vi "SwitchingCommand.vi"(9 "command":i32(ring)=1 items=["Cycle"=1, "Step"=2, "Continue"=3], 10 "HighSpeedEServer":refnum<k24>, 11 "error in (no error)":errorcluster) -> (3 "error out":errorcluster)   [LabVIEW 2021, in "UnderAutomation.Yaskawa.lvlib"]
uses:
  UnderAutomation.Yaskawa.lvlib
  C:/Users/fg/Documents/Yaskawa.vi/LabVIEW_2024/UnderAutomation.Yaskawa/lib/UnderAutomation.Yaskawa.dll
  LabVIEW_2024/UnderAutomation.Yaskawa/lib/UnderAutomation.Yaskawa.dll
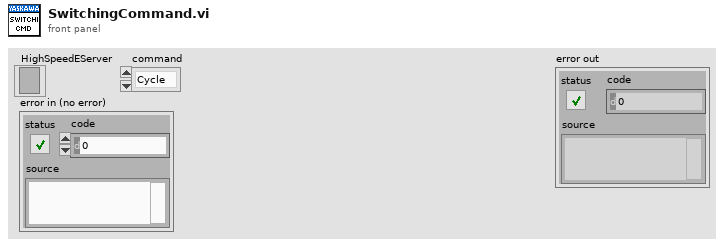
[diagram p1: front panel]
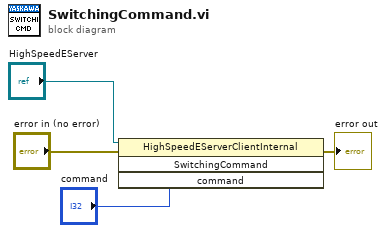
[diagram p0: block diagram]
diagram:
  n1 = invoke class="HighSpeedEServerClientInternal" method="SwitchingCommand"(reference="HighSpeedEServer", error in="error in (no error)", "command"="command") -> (error out=→"error out":errorcluster)  [unwired: 1 in, 3 out]
